vi "List Owned Buckets.vi"() -> ()   [LabVIEW 2011]
doc: "This example demonstrates how you can list the name of the Amazon S3 buckets you own.\n\nTo use this example, <B>you must register with Amazon S3 and have a valid AWS Access Key ID</B> to authenticate requests."
uses:
  Typedefs/Access_Key_Type.ctl
  Typedefs/Secret_Key_Type.ctl
  vi.lib/National Instruments/LabVIEW Interface for Amazon S3/Typedefs/AMZ_S3_AWS Credentials.ctl
  vi.lib/National Instruments/LabVIEW Interface for Amazon S3/LV Interface for Amazon S3.lvlib
panel:
  in  "Secret Key":T1
  in  "Access Key":T2
  out "Buckets":i32(listbox)
  # "To use this VI, you have to register first with Amazon to have an Amazon AWS account.\nIf you don't have an account yet, go to http://aws.amazon.com and Create an AWS account!"
  # "Note: You have to have some buckets created to\nsee any effect after running this VI!\n1. Fill in your AWS Credentials\n2. Run this VI"
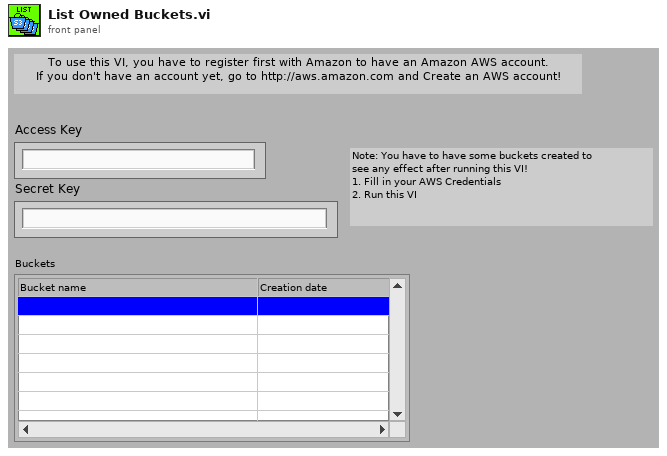
[diagram p1: front panel]
types:
  T1 = typedef "Secret_Key_Type.ctl" = string
  T2 = typedef "Access_Key_Type.ctl" = string
  T3 = typedef "LV Interface for Amazon S3.lvlib/AMZ_S3_AWS Credentials.ctl" = cluster{"Access Key":string, "Secret Key":string}
  T4 = typedef "LV Interface for Amazon S3.lvlib/AMZ_S3_API_Bucket.ctl" = cluster{"Name":string, "CreationDate":timestamp}
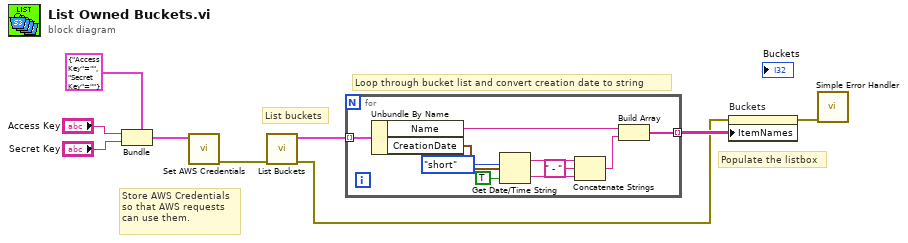
[diagram p0: block diagram]
diagram:
  # "List buckets"
  # "Populate the listbox"
  # "Loop through bucket list and convert creation date to string"
  # "Store AWS Credentials\nso that AWS requests\ncan use them."
  n1 = Bundle(cluster=T3 {"Access Key"="", "Secret Key"=""} ("AWS Credentials in"), "Access Key"="Access Key", "Secret Key"="Secret Key") -> (w1:T3)
  n2 = call "Set AWS Credentials.vi"("AWS Credentials in"=w1) -> ("error out"=w9:errorcluster)  [unwired: 10 in]
  n3 = call "List Buckets.vi"("error in (no error)"=w9) -> ("error out"=w6:errorcluster, "Buckets"=w8:T4[])  [unwired: 9 in]
  n4 = for {
    tunnel: w8 -> [w19] mode=indexing
    tunnel: [w10] -> w7 mode=indexing
    n5 = Unbundle By Name(w19) -> ("Name"=w11:string, "CreationDate"=w18:timestamp)
    n6 = Get Date/Time String(date format (0)=enum16{"short", "long", "abbreviated"}."short", seconds (now)=w18, want seconds? (F)=TRUE) -> (date string=w15:string, time string=w14:string)
    n7 = Concatenate Strings(w15, " - " ("string"), w14) -> (w12:string)
    n8 = Build Array(w11, w12) -> (w10:string[])
  }
  n9 = property on="Buckets" class="MCListbox (strict)"(error in=w6, "ItemNames"=w7) -> (error out=w5:errorcluster)  [unwired: 1 in, 1 out]
  n10 = call <vilib>:"Simple Error Handler.vi"("error in (no error)"=w5) -> ()  [unwired: 4 in, 5 out]
